vi "Plugin.Iteration.Increment.vi"(8 "error in (no error)":errorcluster, 11 "Plugin in":refnum<class "Plugin.lvclass">) -> (0 "error out":errorcluster, 3 "Plugin out":refnum<class "Plugin.lvclass">)   [LabVIEW 2017, in "DSF Core.lvlib" / "Plugin.lvclass"]
uses:
  Plugin.lvclass
  Plugin.lvclass/Plugin.ctl
  Timing/Timing.lvclass/Timing.ctl
  Timing/Timing.lvclass
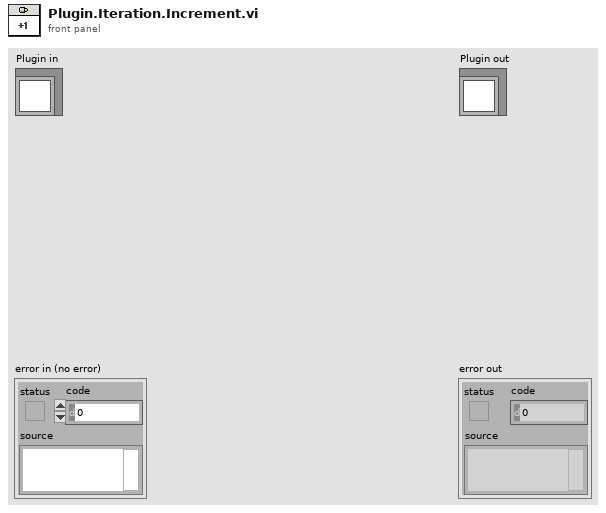
[diagram p1: front panel]
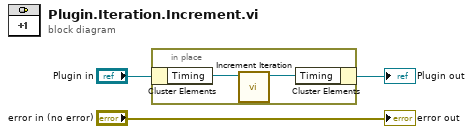
[diagram p0: block diagram]
diagram:
  n1 = in-place {
    n2 = in-place-cluster #1("Plugin in") -> ("Timing"=w5:refnum<class "Timing.lvclass">)
    n3 = call "Increment Iteration.vi"("Timing in"=w5) -> ("Timing out"=w4:refnum<class "Timing.lvclass">)  [unwired: 10 in]
    n4 = in-place-cluster #1("Timing"=w4) -> (→"Plugin out":refnum<class "Plugin.lvclass">)
  }
  "error out" <- "error in (no error)"
